vi "PWM_generation_with_6555.vi"(6 "Phase":dbl format="%0.2f", 7 "Channel List":string="0-2", 8 "error in (no error)":errorcluster, 9 "Duty Cycle":dbl=50.0 format="%.2p", 10 "Frequency":dbl=10000.0 format="%.2p", 11 "Resource Name":refnum<k15>="PXI1Slot7") -> (0 "error out":errorcluster)   [LabVIEW 2016]
doc: "I Description:\nThis example demonstrates how to repeat generation of a dynamic pattern at specified clock rate.\n\nII Instructions for Running:\n1. Browse to the HWS file that you would like to generate. For an example of an HWS file, browse to …\\LabVIEW 7.0\\examples\\instr\\niHSDIO\\Support Files\\Mywfm.hws.\n2. Enter the digital channels on the hardware device to generate digital pattern in the Channel List control.\n3. Specify the clock rate for the generation in the Clock Rate control.\n4. Specify the repeat mode in the Repeat Mode. If Finite is selected, then specify the repeat count in the Repeat Count control. Otherwise, this control is ignored.\n\nIII Block Diagram Steps:\n1. Initialize for a generation session.\n2. Assign specified channels in Channel List for dynamic operation.\n3. Configure the Sample clock to use the onboard clock, and configure the clock rate.\n4. Configure the generation repeat mode.\n5. Query the Data Width property to determine which Write function to use.\nNote: Different devices have different default values for the Data Width property. If you know the Data Width of your device, you may omit the property node and case structure.\n6. Retrieve a digital pattern from an HWS file and write to the onboard memory of the digital device.\n7. Initiate dynamic pattern generation.\n8. Poll to wait for the generation to complete, a click of the stop button, or an error.\n9. Abort generation and close the session.\n\nIV I/O Connections Overview:\nMake connections from output terminals to match the channels specified by Channel List. In this example, a digital pattern is generated from the first 16 digital channels of the device."
uses:
  <instrlib>/niHSDIO/niHSDIO.llb/niHSDIO_ctl Repeat Mode Values (Ring).ctl
  <instrlib>/niHSDIO/niHSDIO.llb/niHSDIO_ctl Sample Clock Source Values (ComboBox).ctl
  <instrlib>/niHSDIO/niHSDIO.llb/niHSDIO_ctl Voltage Logic Family Values (Ring).ctl
  <instrlib>/niHSDIO/niHSDIO.llb/niHSDIO Configure Data Voltage Logic Family.vi
  <instrlib>/niHSDIO/niHSDIO.llb/niHSDIO Write Named Waveform (1D U32).vi
  <vilib>/Analysis/NI_AALBase.lvlib
panel:
  in  "stop":bool
  out "Waveform Graph":u32[](graph)
  out "Loop count":i32
  in  "Repeat Mode":T1=17 items=["Finite"=16, "Continuous"=17]
  in  "Repeat Count":i32=500
  in  "Clock Rate":dbl=1000000.0 format="%.2p"
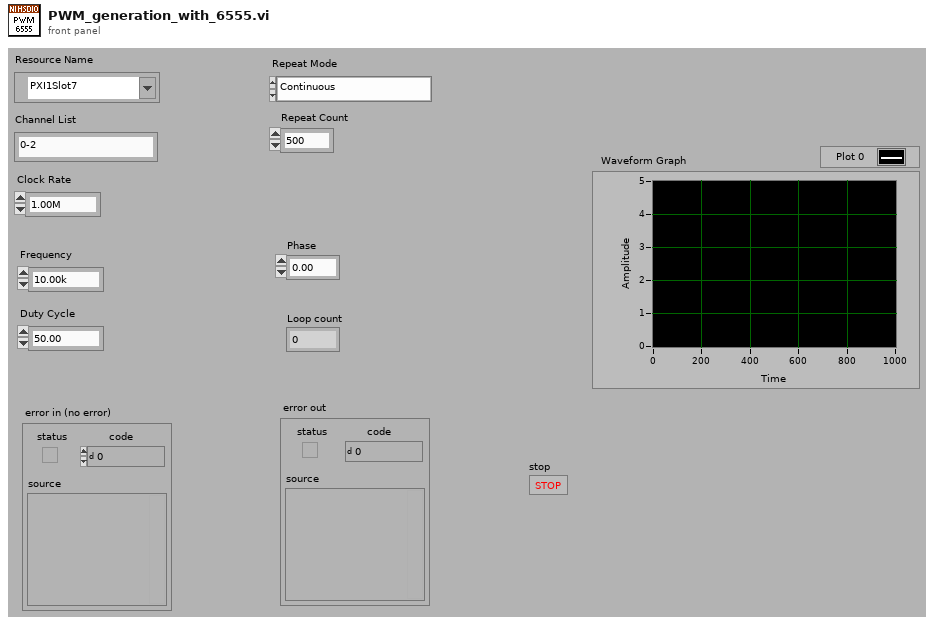
[diagram p1: front panel]
types:
  T1 = typedef "niHSDIO_ctl Repeat Mode Values (Ring).ctl" = i32
  T2 = typedef "niHSDIO_ctl Voltage Logic Family Values (Ring).ctl" = i32
  T3 = typedef "niHSDIO_ctl Sample Clock Source Values (ComboBox).ctl" = string
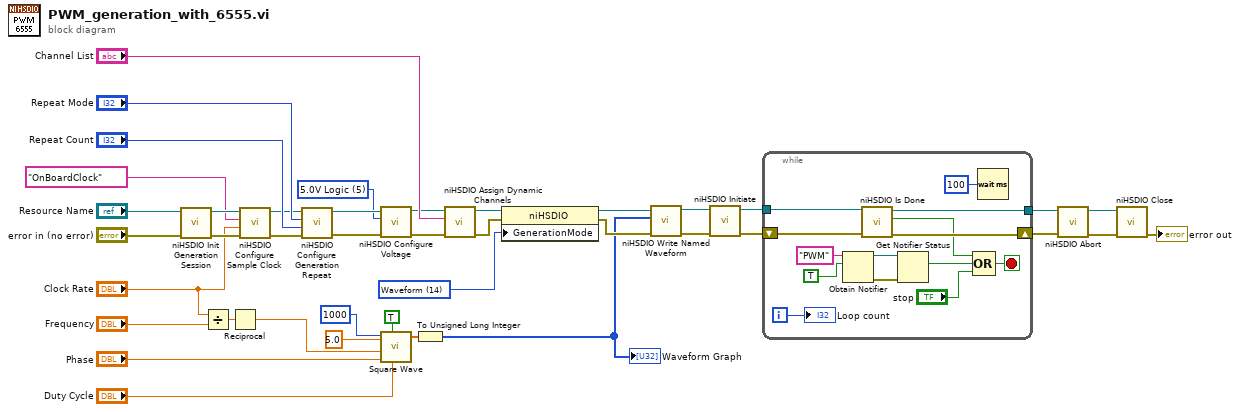
[diagram p0: block diagram]
diagram:
  w6 = 14 items=["Waveform"=14, "Scripted"=15] ("Dynamic Generation:Generation Mode")
  w20 = T2 5 items=["5.0V Logic"=5, "3.3V Logic"=6, "2.5V Logic"=7, "1.8V Logic"=8, "1.5V Logic"=80, "1.2V Logic"=81] ("logic family (3.3V logic)")
  n1 = call <instrlib>:"niHSDIO Init Generation Session.vi"("error in (no error)"="error in (no error)", "resource name"="Resource Name") -> ("error out"=w38:errorcluster, "instrument handle out"=w37:refnum<k15>)  [unwired: 8 in]
  n2 = Divide(x="Clock Rate", y="Frequency") -> (x/y=w10:dbl)
  n3 = Reciprocal(x=w10) -> (1/x=w13:dbl)
  n4 = call <instrlib>:"niHSDIO Configure Sample Clock.vi"("error in (no error)"=w38, "clock rate (50MHz)"="Clock Rate", "clock source (on board clock)"=T3 "OnBoardClock", "instrument handle"=w37) -> ("error out"=w27:errorcluster, "instrument handle out"=w28:refnum<k15>)  [unwired: 6 in]
  n5 = call <instrlib>:"niHSDIO Configure Generation Repeat.vi"("error in (no error)"=w27, "repeat count (1)"="Repeat Count", "repeat mode (finite)"="Repeat Mode", "instrument handle"=w28) -> ("error out"=w19:errorcluster, "instrument handle out"=w21:refnum<k15>)  [unwired: 6 in]
  n6 = call-poly <instrlib>:"niHSDIO Configure Voltage.vi"("error in (no error)"=w19, "logic family (3.3V logic)"=w20, "instrument handle"=w21) -> ("error out"=w9:errorcluster, "instrument handle out"=w7:refnum<k15>)  [unwired: 7 in]
  n7 = call <vilib>:"Square Wave.vi"("samples"=1000, "reset phase"=TRUE, "amplitude"=5.0, "frequency"=w13, "duty cycle (%)"="Duty Cycle", "phase in"="Phase") -> ("square wave"=w24:dbl[])  [unwired: 2 out]
  n8 = To Unsigned Long Integer(number=w24) -> (unsigned 32bit integer=w1:u32[])
  "Waveform Graph" <- w1
  n9 = call <instrlib>:"niHSDIO Assign Dynamic Channels.vi"("error in (no error)"=w9, "channel list (all:\"\")"="Channel List", "instrument handle"=w7) -> ("error out"=w4:errorcluster, "instrument handle out"=w5:refnum<k15>)  [unwired: 7 in]
  n10 = property on="Property Node" class="niHSDIO"(reference=w5, error in=w4, "GenerationMode"=w6) -> (reference out=w3:refnum<k15>, error out=w2:errorcluster)
  n11 = call-poly <instrlib>:"niHSDIO Write Named Waveform.vi"("error in (no error)"=w2, "data"=w1, "instrument handle"=w3) -> ("error out"=w22:errorcluster, "instrument handle out"=w23:refnum<k15>)  [unwired: 7 in]
  n12 = call <instrlib>:"niHSDIO Initiate.vi"("error in (no error)"=w22, "instrument handle"=w23) -> ("error out"=w35:errorcluster, "instrument handle out"=w36:refnum<k15>)  [unwired: 8 in]
  n13 = while {
    tunnel: w36 -> [w54]
    tunnel: [w52] -> w33
    shift-right: [w51] -> w34
    shift-left: w35 -> [w53]
    i -> [w45]
    stop <- w41 stop-if-true
    n14 = Obtain Notifier(name (unnamed)="PWM", notification data type=TRUE) -> (notifier out=w48:refnum<notifier>, error out=w47:errorcluster)  [unwired: 2 in, 1 out]
    n15 = call <instrlib>:"niHSDIO Is Done.vi"("error in (no error)"=w53, "instrument handle"=w54) -> ("error out"=w51:errorcluster, "done"=w44:bool, "instrument handle out"=w52:refnum<k15>)  [unwired: 7 in]
    n16 = Get Notifier Status(notifier=w48, error in (no error)=w47) -> (current notification=w43:bool)  [unwired: 4 out]
    n17 = Compound Arithmetic op=OR(w44, w43, "stop") -> (w41:bool)
    n18 = Wait (ms)(milliseconds to wait=u32 100) -> ()  [unwired: 1 out]
    "Loop count" <- w45
  }
  n19 = call <instrlib>:"niHSDIO Abort.vi"("error in (no error)"=w34, "instrument handle"=w33) -> ("error out"=w31:errorcluster, "instrument handle out"=w32:refnum<k15>)  [unwired: 8 in]
  n20 = call <instrlib>:"niHSDIO Close.vi"("error in (no error)"=w31, "instrument handle"=w32) -> ("error out"=→"error out":errorcluster)  [unwired: 9 in]
